vi "Configure User Defined Event (Range).vi"(0 "VISA resource name":refnum<visa-resource-name>, 2 "Enable User Defined Range Event (T: Enable)":bool=TRUE, 3 "Event Number (1)":i32=1 min=1 max=8 step=1, 5 "Function (Empty)":string, 7 "Judgment Condition 2 (0: OFF)":i32(ring) items=["OFF", "<", "<=", "=", ">", ">=", "!="], 9 "Reference Value 2 (0.0000)":dbl min=-1000000000000.0 max=1000000000000.0 format="%.4g", 11 "error in (no error)":errorcluster, 12 "Judgment Condition 1 (0: OFF)":i32(ring) items=["OFF", "<", "<=", "=", ">", ">=", "!="], 13 "Reference Value 1 (0.0000)":dbl min=-1000000000000.0 max=1000000000000.0 format="%.4g") -> (4 "VISA resource name out":refnum<visa-resource-name>, 15 "error out":errorcluster)   [LabVIEW 2021, in "Yokogawa WT1800 Series.lvlib"]
doc: "Configures the user-defined events features, when the judgment condition specification method is Range.\nSpecify judgment conditions using ranges of measurement function values or differences from a reference value."
uses:
  <instrlib>/Yokogawa WT1800 Series/Yokogawa WT1800 Series.lvlib
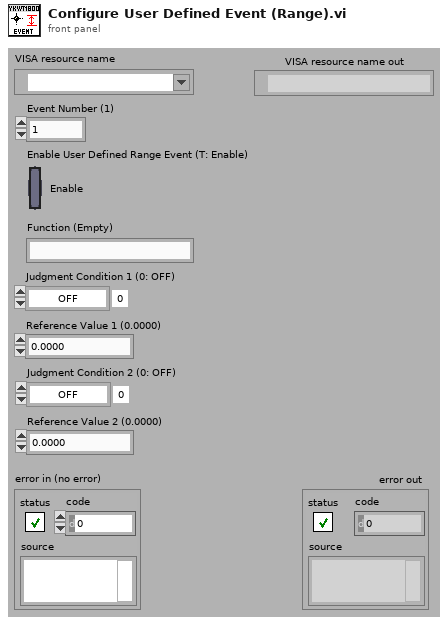
[diagram p1: front panel]
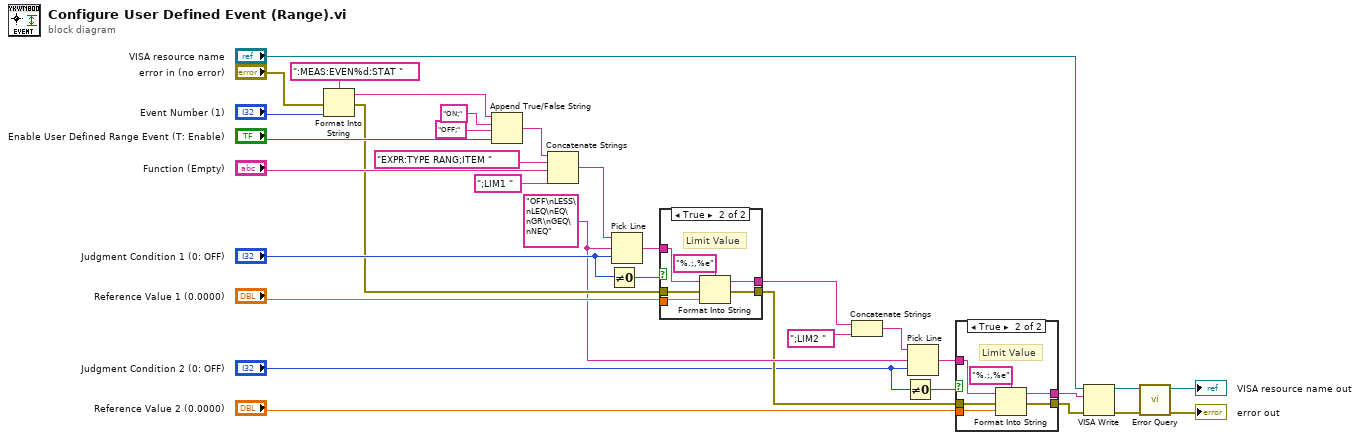
[diagram p0: block diagram]
diagram:
  w6 = "OFF\nLESS\nLEQ\nEQ\nGR\nGEQ\nNEQ" ("複数行文字列")
  n1 = Format Into String(format string=":MEAS:EVEN%d:STAT " ("形式文字列"), error in="error in (no error)", "Event Number (1)") -> (resulting string=w24:string, error out=w12:errorcluster)  [unwired: 1 in]
  n2 = Append True/False String ("True/False 文字列を追加")(1:"Enable User Defined Range Event (T: Enable)", 2:"OFF;", 3:"ON;", 4:w24) -> (0:w21:string)
  n3 = Concatenate Strings(w21, "EXPR:TYPE RANG;ITEM " ("文字列"), "Function (Empty)", ";LIM1 " ("文字列")) -> (w18:string)
  n4 = Not Equal To 0?(x="Judgment Condition 1 (0: OFF)") -> (x != 0?=w16:bool)
  n5 = Pick Line ("ライン選択")(string ("")=w18, multi-line string=w6, line index="Judgment Condition 1 (0: OFF)") -> (output string=w13:string)
  n6 = case shown="True" w16 {
    tunnel: "Reference Value 1 (0.0000)" -> [_ w40]
    tunnel: w13 -> [w35 w39]
    tunnel: w12 -> [w34 w38]
    tunnel: [w35 w37] -> w8
    tunnel: [w34 w36] -> w5
    frame False {
      # "OFF"
    }
    frame True {
      # "Limit Value"
      n7 = Format Into String(format string="%.;,%e" ("形式文字列"), initial string=w39, error in=w38, w40) -> (resulting string=w37:string, error out=w36:errorcluster)
    }
  }
  n8 = Concatenate Strings(w8, ";LIM2 " ("文字列")) -> (w7:string)
  n9 = Not Equal To 0?(x="Judgment Condition 2 (0: OFF)") -> (x != 0?=w10:bool)
  n10 = Pick Line ("ライン選択")(string ("")=w7, multi-line string=w6, line index="Judgment Condition 2 (0: OFF)") -> (output string=w11:string)
  n11 = case shown="True" w10 {
    tunnel: w11 -> [w43 w48]
    tunnel: w5 -> [w42 w47]
    tunnel: "Reference Value 2 (0.0000)" -> [_ w46]
    tunnel: [w43 w45] -> w2
    tunnel: [w42 w44] -> w1
    frame False {
      # "OFF"
    }
    frame True {
      # "Limit Value"
      n12 = Format Into String(format string="%.;,%e" ("形式文字列"), initial string=w48, error in=w47, w46) -> (resulting string=w45:string, error out=w44:errorcluster)
    }
  }
  n13 = VISA Write ("VISA書き込み")(VISA resource name="VISA resource name", write buffer=w2, error in (no error)=w1) -> (VISA resource name out=w33:refnum<visa-resource-name>, error out=w32:errorcluster)  [unwired: 1 out]
  n14 = call <instrlib>:"Error Query.vi"("error in (no error)"=w32, "VISA resource name"=w33) -> ("error out"=→"error out":errorcluster, "VISA resource name out"=→"VISA resource name out":refnum<visa-resource-name>)  [unwired: 6 in, 2 out]
